vi "SMC_GetSt.vi"(8 "error in (no error)":errorcluster) -> (0 "error out":errorcluster, 3 "Answer":string)   [LabVIEW 2015]
uses:
  SMC_SubVIs.llb/SMC_ManagerMode.ctl
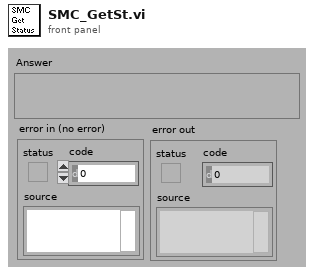
[diagram p1: front panel]
types:
  T1 = typedef "SMC_ManagerMode.ctl" = enum16{"Init", "Get", "SetPosition", "SetStatus", "SetMoving", "SetControllerNr"}
  T2 = typedef "SMC Paras.ctl" = cluster{"VENUS Language":T3, "Number of Axis":u8, "Controller Nr":u8, "Simulation":bool}
  T3 = typedef "VENUSNr.ctl" = enum16{"VENUS 2", "VENUS 1"}
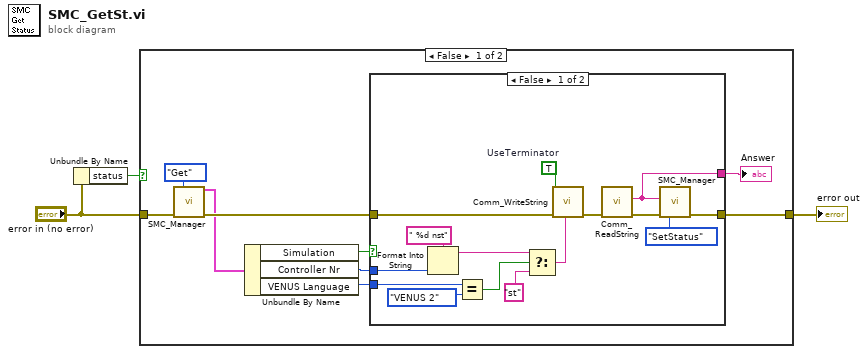
[diagram p0: block diagram]
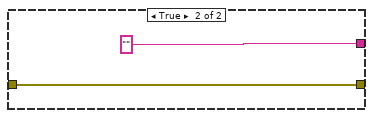
[diagram p2: hidden frame]
diagram:
  n1 = Unbundle By Name("error in (no error)") -> ("status"=w3:bool)
  n2 = case shown="False" w3 {
    tunnel: "error in (no error)" -> [w9 w30]
    tunnel: [w10 w30] -> w1
    frame False {
      n3 = call "SMC_Manager.vi"("Mode"=SMC_ManagerMode."Get", "error in (no error)"=w9) -> ("SMC Parameter Out"=w7:T2, "error out"=w8:errorcluster)  [unwired: 9 in, 3 out]
      n4 = Unbundle By Name(w7) -> ("Simulation"=w4:bool, "Controller Nr"=w5:u8, "VENUS Language"=w6:T3)
      n5 = case shown="False" w4 {
        tunnel: [w21 "" ("Answer")] -> w11
        tunnel: [w26 w29] -> w10
        tunnel: w8 -> [w25 w29]
        tunnel: w6 -> [w20 _]
        tunnel: w5 -> [w14 _]
        frame False {
          w13 = TRUE  # UseTerminator
          n6 = Format Into String(format string=" %d nst" ("Format String"), w14) -> (resulting string=w17:string)  [unwired: 2 in, 1 out]
          n7 = Equal?(x=w20, y=enum16{"VENUS 2", "VENUS 1"}."VENUS 2") -> (x = y?=w18:bool)
          n8 = Select(t=w17, s=w18, f="st" ("string to write")) -> (s? t:f=w15:string)
          n9 = call "Comm_WriteString.vi"("string to write"=w15, "error in (no error)"=w25, "UseTerminator"=w13) -> ("error out"=w22:errorcluster)  [unwired: 8 in]
          n10 = call "Comm_ReadString.vi"("error in (no error)"=w22) -> ("error out"=w24:errorcluster, "Answer"=w21:string)  [unwired: 9 in]
          n11 = call "SMC_Manager.vi"("Mode"=SMC_ManagerMode."SetStatus", "error in (no error)"=w24, "String In"=w21) -> ("error out"=w26:errorcluster)  [unwired: 8 in, 4 out]
        }
        frame True {
        }
      }
      "Answer" <- w11
    }
    frame True {
      # "Error, do nothing"
    }
  }
  "error out" <- w1
